vi "Controls Enable.vi"(8 "Enable/Disable":i32, 11 "Scan Enable/Diable Cluster":T1) -> ()   [LabVIEW 2010]
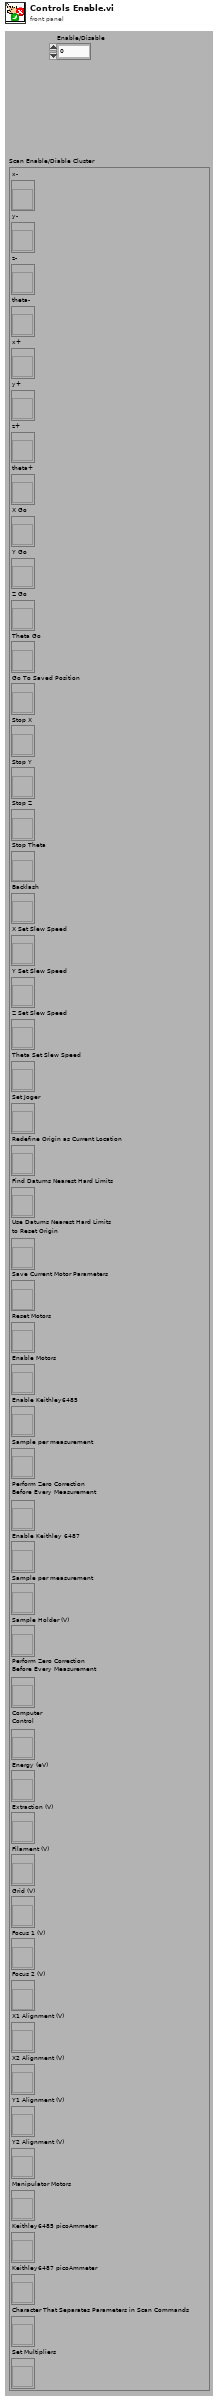
[diagram p1: front panel]
types:
  T1 = cluster{"x-":refnum<vi>, "y-":refnum<vi>, "z-":refnum<vi>, "theta-":refnum<vi>, "x+":refnum<vi>, "y+":refnum<vi>, "z+":refnum<vi>, "theta+":refnum<vi>, "X Go":refnum<vi>, "Y Go":refnum<vi>, "Z Go":refnum<vi>, "Theta Go":refnum<vi>, "Go To Saved Position":refnum<vi>, "Stop X":refnum<vi>, "Stop Y":refnum<vi>, "Stop Z":refnum<vi>, "Stop Theta":refnum<vi>, "Backlash":refnum<vi>, "X Set Slew Speed":refnum<vi>, "Y Set Slew Speed":refnum<vi>, "Z Set Slew Speed":refnum<vi>, "Theta Set Slew Speed":refnum<vi>, "Set Joger":refnum<vi>, "Redefine Origin as Current Location":refnum<vi>, "Find Datums Nearest Hard Limits":refnum<vi>, "Use Datums Nearest Hard Limits\nto Reset Origin":refnum<vi>, "Save Current Motor Parameters":refnum<vi>, "Reset Motors":refnum<vi>, "Enable Motors":refnum<vi>, "Enable Keithley6485":refnum<vi>, "Sample per measurement":refnum<vi>, "Perform Zero Correction\nBefore Every Measurement":refnum<vi>, "Enable Keithley 6487 ":refnum<vi>, "Sample per measurement":refnum<vi>, "Sample Holder (V)":refnum<vi>, "Perform Zero Correction\nBefore Every Measurement":refnum<vi>, "Computer\nControl":refnum<vi>, "Energy (eV)":refnum<vi>, "Extraction (V)":refnum<vi>, "Filament (V)":refnum<vi>, "Grid (V)":refnum<vi>, "Focus 1 (V)":refnum<vi>, "Focus 2 (V)":refnum<vi>, "X1 Alignment (V)":refnum<vi>, "X2 Alignment (V)":refnum<vi>, "Y1 Alignment (V)":refnum<vi>, "Y2 Alignment (V)":refnum<vi>, "Manipulator Motors":refnum<vi>, "Keithley6485 picoAmmeter":refnum<vi>, "Keithley6487 picoAmmeter":refnum<vi>, "Character That Separates Parameters in Scan Commands":refnum<vi>, "Set Multipliers":refnum<vi>}
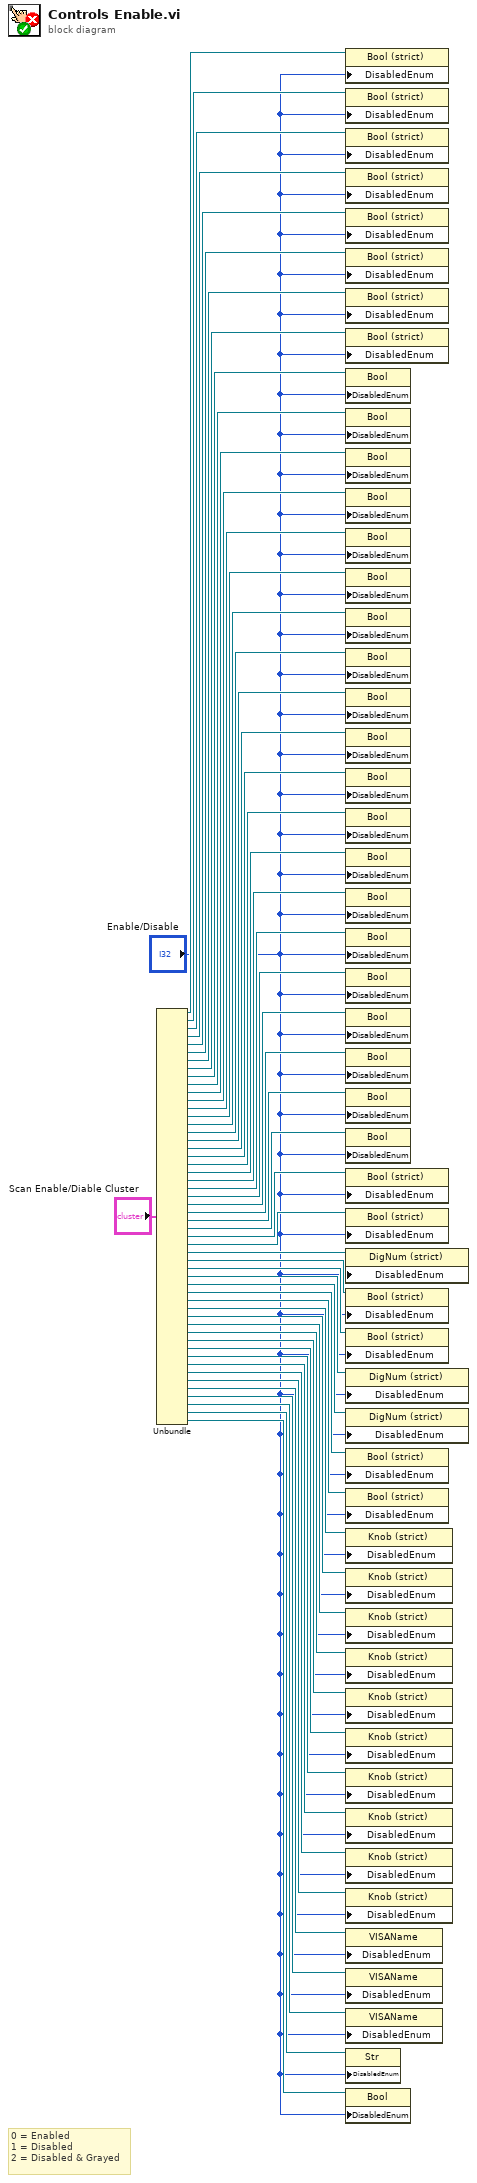
[diagram p0: block diagram]
diagram:
  # "0 = Enabled\n1 = Disabled\n2 = Disabled & Grayed"
  n1 = Unbundle("Scan Enable/Diable Cluster") -> ("x-"=w54:refnum<vi>, "y-"=w53:refnum<vi>, "z-"=w52:refnum<vi>, "theta-"=w51:refnum<vi>, "x+"=w50:refnum<vi>, "y+"=w49:refnum<vi>, "z+"=w48:refnum<vi>, "theta+"=w47:refnum<vi>, "X Go"=w46:refnum<vi>, "Y Go"=w45:refnum<vi>, "Z Go"=w44:refnum<vi>, "Theta Go"=w43:refnum<vi>, "Go To Saved Position"=w42:refnum<vi>, "Stop X"=w41:refnum<vi>, "Stop Y"=w40:refnum<vi>, "Stop Z"=w39:refnum<vi>, "Stop Theta"=w38:refnum<vi>, "Backlash"=w37:refnum<vi>, "X Set Slew Speed"=w36:refnum<vi>, "Y Set Slew Speed"=w35:refnum<vi>, "Z Set Slew Speed"=w34:refnum<vi>, "Theta Set Slew Speed"=w33:refnum<vi>, "Set Joger"=w32:refnum<vi>, "Redefine Origin as Current Location"=w31:refnum<vi>, "Find Datums Nearest Hard Limits"=w30:refnum<vi>, "Use Datums Nearest Hard Limits\nto Reset Origin"=w29:refnum<vi>, "Save Current Motor Parameters"=w28:refnum<vi>, "Reset Motors"=w27:refnum<vi>, "Enable Motors"=w26:refnum<vi>, "Enable Keithley6485"=w25:refnum<vi>, "Sample per measurement"=w24:refnum<vi>, "Perform Zero Correction\nBefore Every Measurement"=w23:refnum<vi>, "Enable Keithley 6487"=w22:refnum<vi>, "Sample per measurement"=w21:refnum<vi>, "Sample Holder (V)"=w20:refnum<vi>, "Perform Zero Correction\nBefore Every Measurement"=w19:refnum<vi>, "Computer\nControl"=w18:refnum<vi>, "Energy (eV)"=w17:refnum<vi>, "Extraction (V)"=w16:refnum<vi>, "Filament (V)"=w15:refnum<vi>, "Grid (V)"=w14:refnum<vi>, "Focus 1 (V)"=w13:refnum<vi>, "Focus 2 (V)"=w12:refnum<vi>, "X1 Alignment (V)"=w11:refnum<vi>, "X2 Alignment (V)"=w10:refnum<vi>, "Y1 Alignment (V)"=w9:refnum<vi>, "Y2 Alignment (V)"=w8:refnum<vi>, "Manipulator Motors"=w7:refnum<vi>, "Keithley6485 picoAmmeter"=w6:refnum<vi>, "Keithley6487 picoAmmeter"=w5:refnum<vi>, "Character That Separates Parameters in Scan Commands"=w4:refnum<vi>, "Set Multipliers"=w2:refnum<vi>)
  n2 = property class="Bool (strict)"(reference=w54, "DisabledEnum"="Enable/Disable") -> ()  [unwired: 1 in, 2 out]
  n3 = property class="Bool (strict)"(reference=w53, "DisabledEnum"="Enable/Disable") -> ()  [unwired: 1 in, 2 out]
  n4 = property class="Bool (strict)"(reference=w52, "DisabledEnum"="Enable/Disable") -> ()  [unwired: 1 in, 2 out]
  n5 = property class="Bool (strict)"(reference=w51, "DisabledEnum"="Enable/Disable") -> ()  [unwired: 1 in, 2 out]
  n6 = property class="Bool (strict)"(reference=w50, "DisabledEnum"="Enable/Disable") -> ()  [unwired: 1 in, 2 out]
  n7 = property class="Bool (strict)"(reference=w49, "DisabledEnum"="Enable/Disable") -> ()  [unwired: 1 in, 2 out]
  n8 = property class="Bool (strict)"(reference=w48, "DisabledEnum"="Enable/Disable") -> ()  [unwired: 1 in, 2 out]
  n9 = property class="Bool (strict)"(reference=w47, "DisabledEnum"="Enable/Disable") -> ()  [unwired: 1 in, 2 out]
  n10 = property class="Bool"(reference=w46, "DisabledEnum"="Enable/Disable") -> ()  [unwired: 1 in, 2 out]
  n11 = property class="Bool"(reference=w45, "DisabledEnum"="Enable/Disable") -> ()  [unwired: 1 in, 2 out]
  n12 = property class="Bool"(reference=w44, "DisabledEnum"="Enable/Disable") -> ()  [unwired: 1 in, 2 out]
  n13 = property class="Bool"(reference=w43, "DisabledEnum"="Enable/Disable") -> ()  [unwired: 1 in, 2 out]
  n14 = property class="Bool"(reference=w42, "DisabledEnum"="Enable/Disable") -> ()  [unwired: 1 in, 2 out]
  n15 = property class="Bool"(reference=w41, "DisabledEnum"="Enable/Disable") -> ()  [unwired: 1 in, 2 out]
  n16 = property class="Bool"(reference=w40, "DisabledEnum"="Enable/Disable") -> ()  [unwired: 1 in, 2 out]
  n17 = property class="Bool"(reference=w39, "DisabledEnum"="Enable/Disable") -> ()  [unwired: 1 in, 2 out]
  n18 = property class="Bool"(reference=w38, "DisabledEnum"="Enable/Disable") -> ()  [unwired: 1 in, 2 out]
  n19 = property class="Bool"(reference=w37, "DisabledEnum"="Enable/Disable") -> ()  [unwired: 1 in, 2 out]
  n20 = property class="Bool"(reference=w36, "DisabledEnum"="Enable/Disable") -> ()  [unwired: 1 in, 2 out]
  n21 = property class="Bool"(reference=w35, "DisabledEnum"="Enable/Disable") -> ()  [unwired: 1 in, 2 out]
  n22 = property class="Bool"(reference=w34, "DisabledEnum"="Enable/Disable") -> ()  [unwired: 1 in, 2 out]
  n23 = property class="Bool"(reference=w33, "DisabledEnum"="Enable/Disable") -> ()  [unwired: 1 in, 2 out]
  n24 = property class="Bool"(reference=w32, "DisabledEnum"="Enable/Disable") -> ()  [unwired: 1 in, 2 out]
  n25 = property class="Bool"(reference=w31, "DisabledEnum"="Enable/Disable") -> ()  [unwired: 1 in, 2 out]
  n26 = property class="Bool"(reference=w30, "DisabledEnum"="Enable/Disable") -> ()  [unwired: 1 in, 2 out]
  n27 = property class="Bool"(reference=w29, "DisabledEnum"="Enable/Disable") -> ()  [unwired: 1 in, 2 out]
  n28 = property class="Bool"(reference=w28, "DisabledEnum"="Enable/Disable") -> ()  [unwired: 1 in, 2 out]
  n29 = property class="Bool"(reference=w27, "DisabledEnum"="Enable/Disable") -> ()  [unwired: 1 in, 2 out]
  n30 = property class="Bool (strict)"(reference=w26, "DisabledEnum"="Enable/Disable") -> ()  [unwired: 1 in, 2 out]
  n31 = property class="Bool (strict)"(reference=w25, "DisabledEnum"="Enable/Disable") -> ()  [unwired: 1 in, 2 out]
  n32 = property class="DigNum (strict)"(reference=w24, "DisabledEnum"="Enable/Disable") -> ()  [unwired: 1 in, 2 out]
  n33 = property class="Bool (strict)"(reference=w23, "DisabledEnum"="Enable/Disable") -> ()  [unwired: 1 in, 2 out]
  n34 = property class="Bool (strict)"(reference=w22, "DisabledEnum"="Enable/Disable") -> ()  [unwired: 1 in, 2 out]
  n35 = property class="DigNum (strict)"(reference=w21, "DisabledEnum"="Enable/Disable") -> ()  [unwired: 1 in, 2 out]
  n36 = property class="DigNum (strict)"(reference=w20, "DisabledEnum"="Enable/Disable") -> ()  [unwired: 1 in, 2 out]
  n37 = property class="Bool (strict)"(reference=w19, "DisabledEnum"="Enable/Disable") -> ()  [unwired: 1 in, 2 out]
  n38 = property class="Bool (strict)"(reference=w18, "DisabledEnum"="Enable/Disable") -> ()  [unwired: 1 in, 2 out]
  n39 = property class="Knob (strict)"(reference=w17, "DisabledEnum"="Enable/Disable") -> ()  [unwired: 1 in, 2 out]
  n40 = property class="Knob (strict)"(reference=w16, "DisabledEnum"="Enable/Disable") -> ()  [unwired: 1 in, 2 out]
  n41 = property class="Knob (strict)"(reference=w15, "DisabledEnum"="Enable/Disable") -> ()  [unwired: 1 in, 2 out]
  n42 = property class="Knob (strict)"(reference=w14, "DisabledEnum"="Enable/Disable") -> ()  [unwired: 1 in, 2 out]
  n43 = property class="Knob (strict)"(reference=w13, "DisabledEnum"="Enable/Disable") -> ()  [unwired: 1 in, 2 out]
  n44 = property class="Knob (strict)"(reference=w12, "DisabledEnum"="Enable/Disable") -> ()  [unwired: 1 in, 2 out]
  n45 = property class="Knob (strict)"(reference=w11, "DisabledEnum"="Enable/Disable") -> ()  [unwired: 1 in, 2 out]
  n46 = property class="Knob (strict)"(reference=w10, "DisabledEnum"="Enable/Disable") -> ()  [unwired: 1 in, 2 out]
  n47 = property class="Knob (strict)"(reference=w9, "DisabledEnum"="Enable/Disable") -> ()  [unwired: 1 in, 2 out]
  n48 = property class="Knob (strict)"(reference=w8, "DisabledEnum"="Enable/Disable") -> ()  [unwired: 1 in, 2 out]
  n49 = property class="VISAName"(reference=w7, "DisabledEnum"="Enable/Disable") -> ()  [unwired: 1 in, 2 out]
  n50 = property class="VISAName"(reference=w6, "DisabledEnum"="Enable/Disable") -> ()  [unwired: 1 in, 2 out]
  n51 = property class="VISAName"(reference=w5, "DisabledEnum"="Enable/Disable") -> ()  [unwired: 1 in, 2 out]
  n52 = property class="Str"(reference=w4, "DisabledEnum"="Enable/Disable") -> ()  [unwired: 1 in, 2 out]
  n53 = property class="Bool"(reference=w2, "DisabledEnum"="Enable/Disable") -> ()  [unwired: 1 in, 2 out]
